vi "DBL-round to p decimal places.vi"(8 "Error In":errorcluster, 10 "p = desired precision = number of digits after decimal point (dflt=2)":u32=2, 11 "x = number in":dbl=1.23456789 format="%.10g") -> (0 "Error Out":errorcluster, 2 "Number out (rounded to p digits after decimal point)":string, 3 "x= number out (rounded to p digits after decimal point)":dbl format="%.10g")   [LabVIEW 2021, in "Numeric Utilities.lvlib"]
uses:
  Numeric Utilities.lvlib
panel:
  out "step 3":dbl format="%.10g"
  out "step 2":dbl format="%.10g"
  out "step 1":dbl format="%.10g"
  # "Development\ncontrols/indicators useful for development and testing, but which are not outputs of the VI"
  # "Input\nInputs to the VI"
  # "Output\nOutputs of the VI"
  # "Description\n\nBlank VI with error handling case. \n\nSummarize the use of this VI in this space."
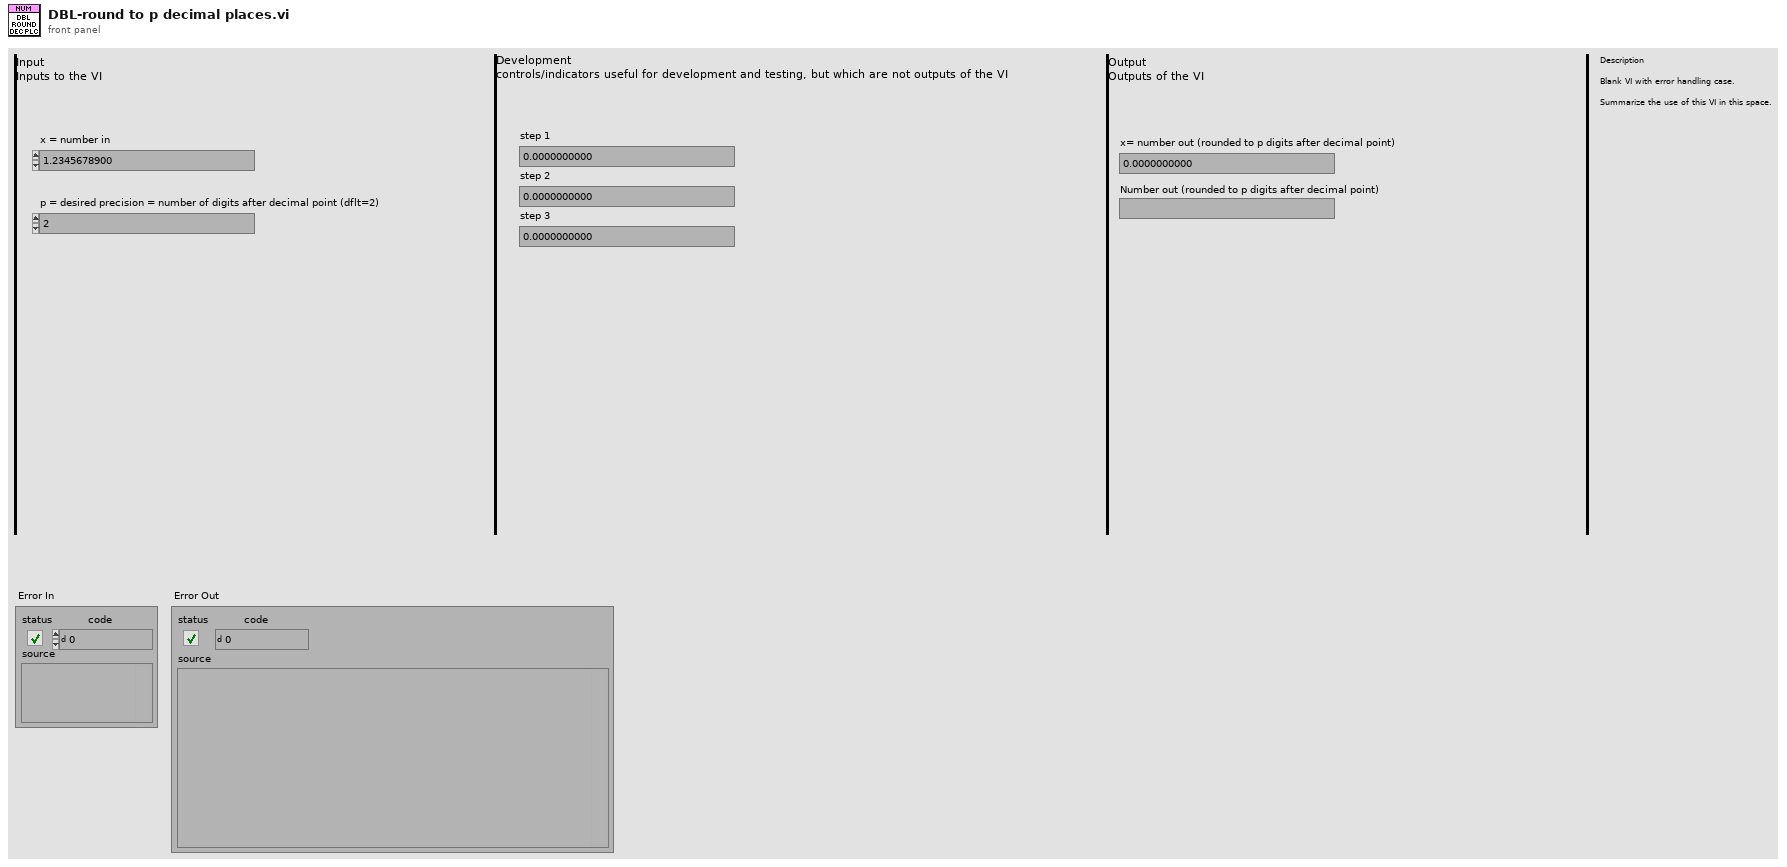
[diagram p1: front panel]
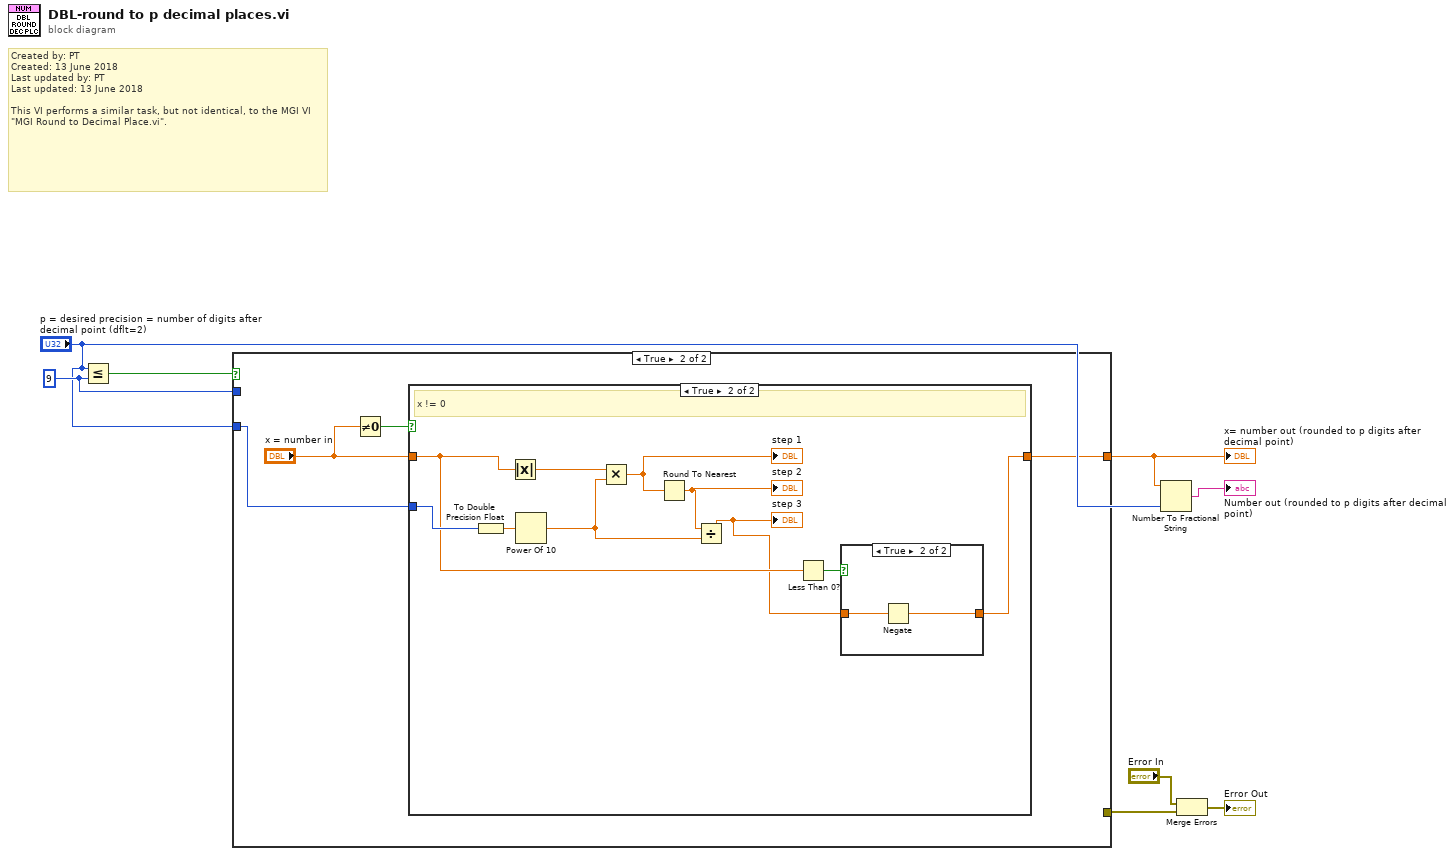
[diagram p0: block diagram]
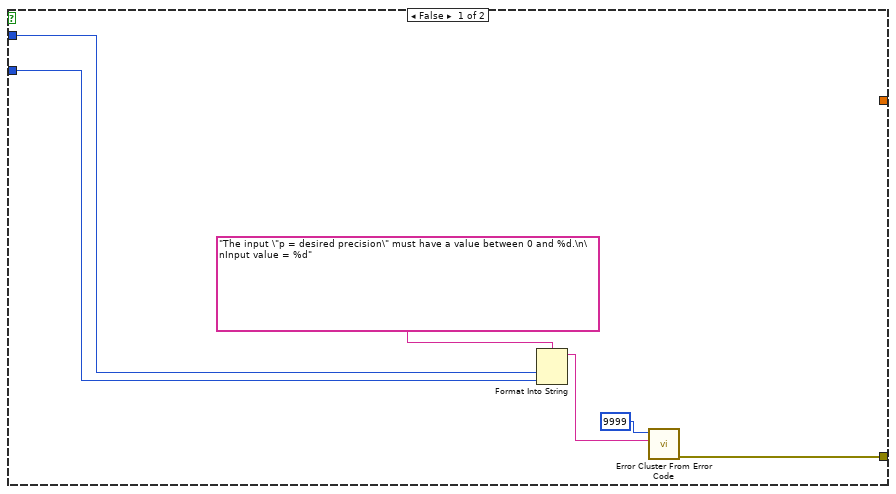
[diagram p2: hidden frame]
diagram:
  w4 = u32 9 ("y")
  # "Created by: PT\nCreated: 13 June 2018\nLast updated by: PT\nLast updated: 13 June 2018\n\nThis VI performs a similar task, but not identical, to the MGI VI \"MGI Round to Decimal Place.vi\"."
  n1 = Less Or Equal?(x="p = desired precision = number of digits after decimal point (dflt=2)", y=w4) -> (x <= y?=w8:bool)
  n2 = case shown="True" w8 {
    tunnel: [w11 _] -> w7
    tunnel: w4 -> [w14 _]
    tunnel: "p = desired precision = number of digits after decimal point (dflt=2)" -> [w13 w15]
    tunnel: [_ w17] -> w3
    frame False {
      n3 = Format Into String(format string="The input \"p = desired precision\" must have a value between 0 and %d.\n\nInput value = %d" ("initial string"), w14, w13) -> (resulting string=w10:string)  [unwired: 2 in, 1 out]
      n4 = call <vilib>:"Error Cluster From Error Code.vi"("error message (\"\")"=w10, "error code (0)"=9999) -> ("error out"=w11:errorcluster)  [unwired: 7 in]
    }
    frame True {
      n5 = Not Equal To 0?(x="x = number in") -> (x != 0?=w18:bool)
      n6 = case shown="True" w18 {
        tunnel: [w19 w20] -> w17
        tunnel: "x = number in" -> [w19 w23]
        tunnel: w15 -> [_ w28]
        frame False {
          # "x == 0"
        }
        frame True {
          # "x != 0"
          n7 = To Double Precision Float(number=w28) -> (double precision float=w27:dbl)
          n8 = Absolute Value(x=w23) -> (abs(x)=w29:dbl)
          n9 = Power Of 10(x=w27) -> (10^x=w24:dbl)
          n10 = Multiply(x=w29, y=w24) -> (x*y=w26:dbl)
          "step 1" <- w26
          n11 = Round To Nearest(number=w26) -> (nearest integer value=w25:dbl)
          "step 2" <- w25
          n12 = Divide(x=w25, y=w24) -> (x/y=w21:dbl)
          "step 3" <- w21
          n13 = Less Than 0?(x=w23) -> (x < 0?=w22:bool)
          n14 = case shown="True" w22 {
            tunnel: w21 -> [w30 w32]
            tunnel: [w30 w31] -> w20
            frame False {
            }
            frame True {
              n15 = Negate(x=w32) -> (-x=w31:dbl)
            }
          }
        }
      }
    }
  }
  "x= number out (rounded to p digits after decimal point)" <- w3
  n16 = Number To Fractional String(number=w3, precision (6)="p = desired precision = number of digits after decimal point (dflt=2)") -> (F-format string=→"Number out (rounded to p digits after decimal point)":string)  [unwired: 2 in]
  n17 = Merge Errors("Error In", w7) -> (→"Error Out":errorcluster)
